vi "SubVi Json GET.vi"(8 "error in (no error)":errorcluster, 9 "input cluster":T2, 10 "Parameter Name All":string="formInput", 11 "Response Body":string) -> (0 "error out":errorcluster, 3 "Cluster":T1)   [LabVIEW 2017]
uses:
  <vilib>/LVH/i3 JSON/JSON Parsing/Get Object Parameter Files/Get Object Parameter - Object.vi
  <vilib>/LVH/i3 JSON/i3-json.lvlib
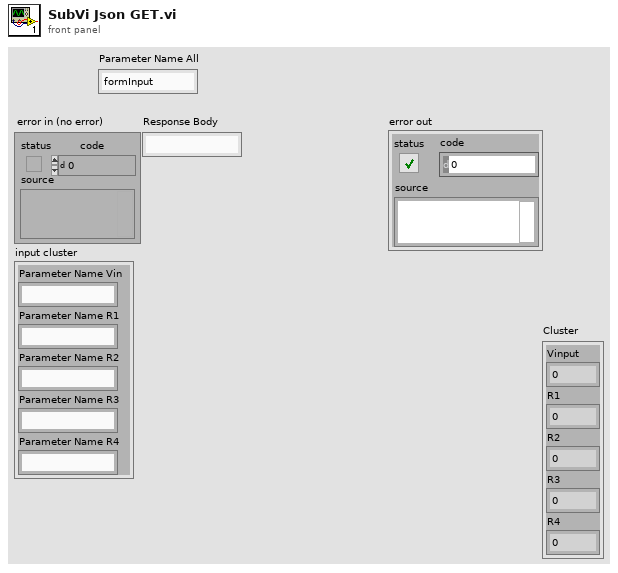
[diagram p1: front panel]
types:
  T1 = cluster{"Vinput":dbl, "R1":dbl, "R2":dbl, "R3":dbl, "R4":dbl}
  T2 = cluster{"Parameter Name Vin":string, "Parameter Name R1":string, "Parameter Name R2":string, "Parameter Name R3":string, "Parameter Name R4":string}
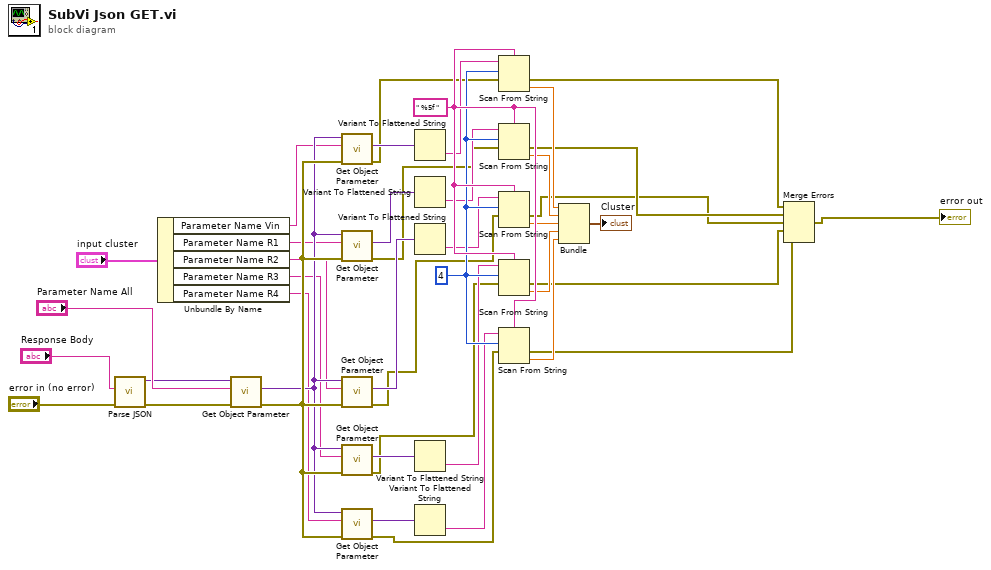
[diagram p0: block diagram]
diagram:
  w22 = u32 4 ("initial scan location")
  w23 = " %5f " ("format string")
  n1 = call <vilib>:"Parse JSON.vi"("error in (no error)"="error in (no error)", "JSON String"="Response Body") -> ("error out"=w39:errorcluster, "JSON Tree"=w41:variant)  [unwired: 6 in, 2 out]
  n2 = Unbundle By Name("input cluster") -> ("Parameter Name Vin"=w34:string, "Parameter Name R1"=w33:string, "Parameter Name R2"=w32:string, "Parameter Name R3"=w31:string, "Parameter Name R4"=w30:string)
  n3 = call-poly <vilib>:"Get Object Parameter.vi"("error in (no error)"=w39, "Parameter Name"="Parameter Name All", "JSON Tree In (JSON Object)"=w41) -> ("error out"=w36:errorcluster, "JSON Object"=w35:variant)  [unwired: 5 in, 2 out]
  n4 = call-poly <vilib>:"Get Object Parameter.vi"("error in (no error)"=w36, "Parameter Name"=w34, "JSON Tree In (JSON Object)"=w35) -> ("error out"=w10:errorcluster, "JSON Object"=w24:variant)  [unwired: 5 in, 2 out]
  n5 = call-poly <vilib>:"Get Object Parameter.vi"("error in (no error)"=w36, "Parameter Name"=w33, "JSON Tree In (JSON Object)"=w35) -> ("error out"=w9:errorcluster, "JSON Object"=w25:variant)  [unwired: 5 in, 2 out]
  n6 = call-poly <vilib>:"Get Object Parameter.vi"("error in (no error)"=w36, "Parameter Name"=w32, "JSON Tree In (JSON Object)"=w35) -> ("error out"=w8:errorcluster, "JSON Object"=w26:variant)  [unwired: 5 in, 2 out]
  n7 = call-poly <vilib>:"Get Object Parameter.vi"("error in (no error)"=w36, "Parameter Name"=w31, "JSON Tree In (JSON Object)"=w35) -> ("error out"=w7:errorcluster, "JSON Object"=w27:variant)  [unwired: 5 in, 2 out]
  n8 = call-poly <vilib>:"Get Object Parameter.vi"("error in (no error)"=w36, "Parameter Name"=w30, "JSON Tree In (JSON Object)"=w35) -> ("error out"=w6:errorcluster, "JSON Object"=w28:variant)  [unwired: 5 in, 2 out]
  n9 = Variant To Flattened String(Variant=w24) -> (data string=w21:string)  [unwired: 1 out]
  n10 = Variant To Flattened String(Variant=w25) -> (data string=w20:string)  [unwired: 1 out]
  n11 = Variant To Flattened String(Variant=w26) -> (data string=w19:string)  [unwired: 1 out]
  n12 = Variant To Flattened String(Variant=w27) -> (data string=w18:string)  [unwired: 1 out]
  n13 = Variant To Flattened String(Variant=w28) -> (data string=w17:string)  [unwired: 1 out]
  n14 = Scan From String(format string=w23, input string=w21, initial scan location=w22, error in=w10) -> (error out=w5:errorcluster, output 1=w15:dbl)  [unwired: 1 in, 2 out]
  n15 = Scan From String(format string=w23, input string=w20, initial scan location=w22, error in=w9) -> (error out=w4:errorcluster, output 1=w14:dbl)  [unwired: 1 in, 2 out]
  n16 = Scan From String(format string=w23, input string=w19, initial scan location=w22, error in=w8) -> (error out=w3:errorcluster, output 1=w13:dbl)  [unwired: 1 in, 2 out]
  n17 = Scan From String(format string=w23, input string=w18, initial scan location=w22, error in=w7) -> (error out=w2:errorcluster, output 1=w12:dbl)  [unwired: 1 in, 2 out]
  n18 = Scan From String(format string=w23, input string=w17, initial scan location=w22, error in=w6) -> (error out=w1:errorcluster, output 1=w11:dbl)  [unwired: 1 in, 2 out]
  n19 = Bundle(w15, w14, w13, w12, w11) -> (→"Cluster":cluster{dbl, dbl, dbl, dbl, dbl})  [unwired: 1 in]
  n20 = Merge Errors(w5, w4, w3, w2, w1) -> (→"error out":errorcluster)
